vi "API Stream Test.vi"() -> ()   [LabVIEW 2019]
uses:
  PF_API.lvclass
panel:
  in  "Select Samples Per Scan":T1(ring)
  in  "UDP Streaming Options":T2
  in  "UDP Streaming Port":u16=61557
  out "Polar Plot":picture
  in  "stop":bool
  in  "Scanner IP Address":string="10.48.0.72"
  in  "Host IP Address":string="10.48.0.61"
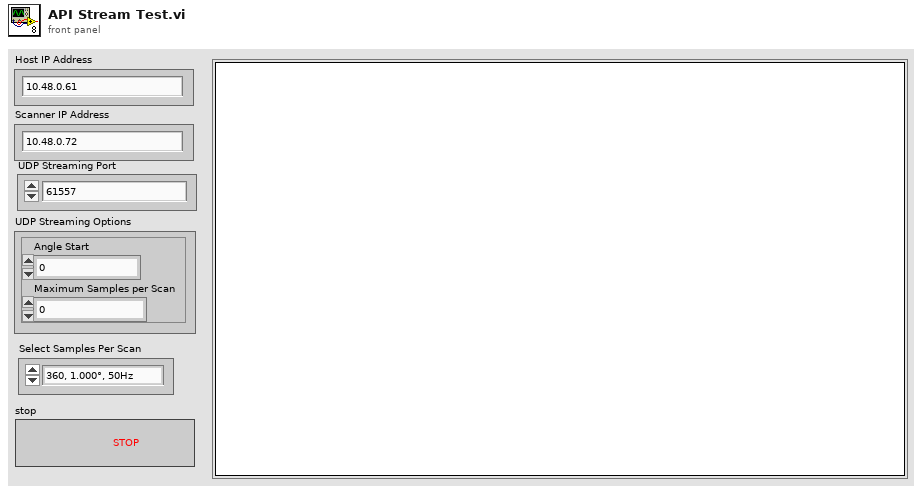
[diagram p1: front panel]
types:
  T1 = enum16{"360, 1.000°, 50Hz", "720, 0.500°, 50Hz", "1440, 0.250°, 50Hz", "360, 1.000°, 35Hz", "720, 0.500°, 35Hz", "1440, 0.250°, 35Hz", "360, 1.000°, 10Hz", "720, 0.500°, 10Hz", "1440, 0.250°, 10Hz"}
  T2 = cluster{"Angle Start":i32, "Maximum Samples per Scan":u16}
  T3 = typedef "LVBoundsTypeDef.ctl" = cluster{"Width":u32, "Height":u32}
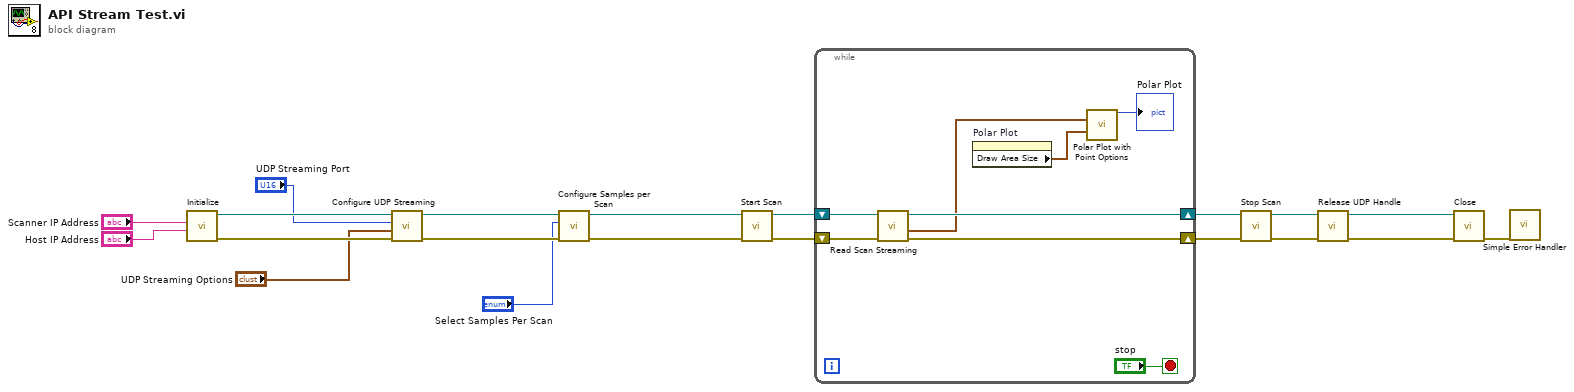
[diagram p0: block diagram]
diagram:
  n1 = call "Initialize.vi"("Host IP Address"="Host IP Address", "Scanner IP Address"="Scanner IP Address") -> ("error out"=w18:errorcluster, "PF_API out"=w17:refnum<class "PF_API.lvclass">)  [unwired: 8 in]
  n2 = call-dynamic "Configure UDP Streaming.vi"("error in (no error)"=w18, "UDP Streaming Options"="UDP Streaming Options", "UDP Streaming Port"="UDP Streaming Port", "PF_API in"=w17) -> ("error out"=w16:errorcluster, "PF_API out"=w5:refnum<class "PF_API.lvclass">)  [unwired: 6 in]
  n3 = call-dynamic "Configure Samples per Scan.vi"("error in (no error)"=w16, "Select Samples Per Scan"="Select Samples Per Scan", "PF_API in"=w5) -> ("error out"=w6:errorcluster, "PF_API out"=w4:refnum<class "PF_API.lvclass">)  [unwired: 7 in]
  n4 = call-dynamic "Start Scan.vi"("error in (no error)"=w6, "PF_API in"=w4) -> ("error out"=w14:errorcluster, "PF_API out"=w15:refnum<class "PF_API.lvclass">)  [unwired: 8 in]
  n5 = while {
    shift-right: [w26] -> w13
    shift-left: w15 -> [w28]
    shift-right: [w25] -> w12
    shift-left: w14 -> [w27]
    stop <- "stop" stop-if-true
    n6 = call-dynamic "Read Scan Streaming.vi"("error in (no error)"=w27, "PF_API in"=w28) -> ("error out"=w25:errorcluster, "Distance x Angle"=w21:cluster{"Magnitude":dbl, "Phase":dbl}[], "PF_API out"=w26:refnum<class "PF_API.lvclass">)  [unwired: 7 in]
    n7 = property on="Polar Plot" class="Pict"() -> ("Draw Area Size"=w23:T3)  [unwired: 2 in, 2 out]
    n8 = call <vilib>:"Polar Plot with Point Options.vi"("data array [mag, phase (deg)]"=w21, "dimensions (w,h)"=w23) -> ("new picture"=→"Polar Plot":picture)  [unwired: 13 in]
  }
  n9 = call-dynamic "Stop Scan.vi"("error in (no error)"=w12, "PF_API in"=w13) -> ("error out"=w10:errorcluster, "PF_API out"=w11:refnum<class "PF_API.lvclass">)  [unwired: 8 in]
  n10 = call-dynamic "Release UDP Handle.vi"("error in (no error)"=w10, "PF_API in"=w11) -> ("error out"=w7:errorcluster, "PF_API out"=w1:refnum<class "PF_API.lvclass">)  [unwired: 8 in]
  n11 = call-dynamic "Close.vi"("error in (no error)"=w7, "PF_API in"=w1) -> ("error out"=w2:errorcluster)  [unwired: 8 in, 1 out]
  n12 = call <vilib>:"Simple Error Handler.vi"("error in (no error)"=w2) -> ()  [unwired: 4 in, 5 out]
